vi "State-Space.vi"(0 "input points":dbl[](array[numeric]) format="%.2f", 1 "initial conditions":dbl[](array[numeric]) format="%.2f", 2 "MIMO state space":T1 {"D" format="%.2f"; "C" format="%.2f"; "B" format="%.2f"; "A" format="%.2f"}, 3 "dt":dbl=1e-09 min=1e-09 format="%.6f", 4 "initialize":bool) -> (5 "output points":dbl[](array[numeric]) format="%.2f", 6 "states":dbl[](array[numeric]) format="%.2f")   [LabVIEW 2020, in "NI_AdvCtrl_continuous linear.lvlib"]
doc: "LabVIEW no longer supports this VI. You can obtain similar functionality by installing the LabVIEW Simulation Module.\n\nCalculates the new output and the internal states, where the state-space representation, the initial condition, and the input vectors are given. The MIMO system is represented by dx(t)/dt=Ax(t)+Bu(t), y(t)=Cx(t)+Du(t)."
uses:
  <vilib>/addons/control/advanced/NI_AdvCtrl_continuous linear.lvlib
  <vilib>/addons/control/advanced/continuous linear.llb/Integrator (DBL Array).vi
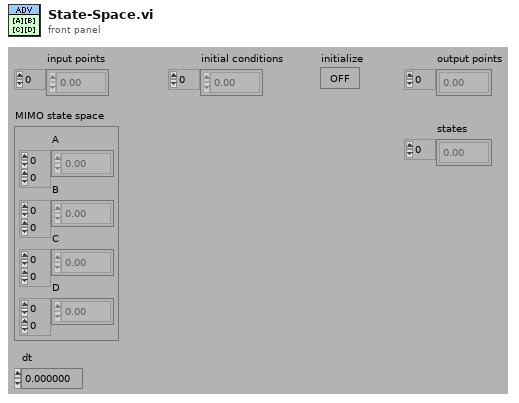
[diagram p1: front panel]
types:
  T1 = cluster{"A":dbl[][], "B":dbl[][], "C":dbl[][], "D":dbl[][]}
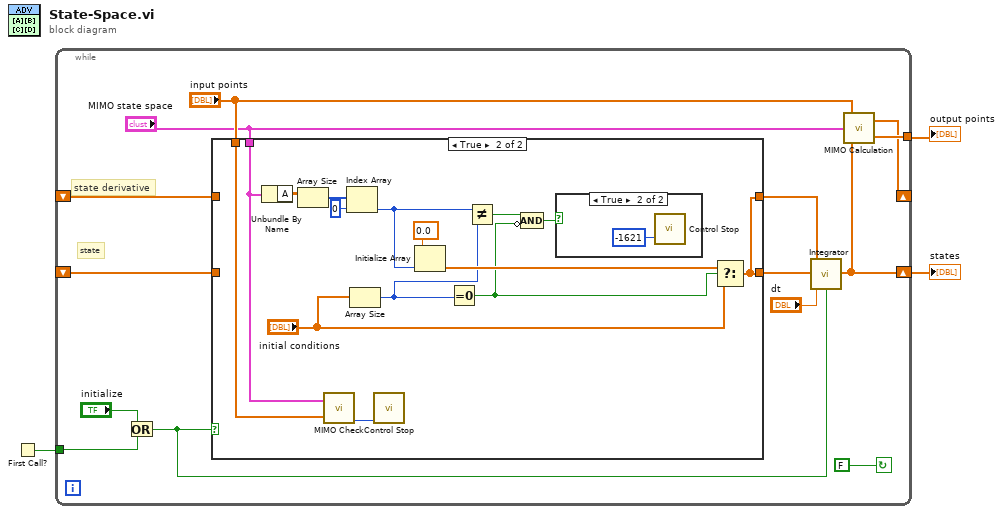
[diagram p0: block diagram]
diagram:
  n1 = First Call?() -> (First Call?: T/F=w1:bool)
  n2 = while {
    tunnel: w1 -> [w8]
    shift-left: _ -> [w14]
    shift-right: [w15] -> _
    tunnel: [w17] -> w3
    shift-left: _ -> [w16]
    shift-right: [w12] -> w2
    stop <- FALSE continue-if-true
    # "state"
    # "state derivative"
    n3 = Or(x="initialize", y=w8) -> (x .or. y?=w6:bool)
    n4 = case shown="True" w6 {
      tunnel: [w19 w20] -> w4
      tunnel: w16 -> [w19 _]
      tunnel: w14 -> [w18 _]
      tunnel: [w18 w20] -> w13
      tunnel: "input points" -> [_ w22]
      tunnel: "MIMO state space" -> [_ w28]
      frame False {
      }
      frame True {
        n5 = Unbundle By Name(w28) -> ("A"=w34:dbl[][])
        n6 = Array Size(array=w34) -> (size(s)=w32:i32[])
        n7 = call <vilib>:"MIMO Check.vi"("MIMO State-Space"=w28, "Input Points"=w22) -> ("error"=w27:i32)  [unwired: 3 out]
        n8 = Index Array(array=w32, index=0 ("Index")) -> (element=w21:i32)
        n9 = Array Size(array="initial conditions") -> (size(s)=w24:i32)
        n10 = call <vilib>:"Control Stop.vi"("error"=w27) -> ()  [unwired: 2 out]
        n11 = Initialize Array(0.0 ("Element Data"), w21) -> (w29:dbl[])
        n12 = Equal To 0?(x=w24) -> (x = 0?=w26:bool)
        n13 = Not Equal?(x=w21, y=w24) -> (x != y?=w25:bool)
        n14 = Compound Arithmetic op=AND(w25, invert w26) -> (w23:bool)
        n15 = case shown="True" w23 {
          frame False {
          }
          frame True {
            n16 = call <vilib>:"Control Stop.vi"("error"=-1621) -> ()  [unwired: 2 out]
          }
        }
        n17 = Select(t=w29, s=w26, f="initial conditions") -> (s? t:f=w20:dbl[])
      }
    }
    n18 = call-poly <vilib>:"Integrator.vi"("initialize"=w6, "dt"="dt", "initial conditions"=w4, "input points"=w13) -> ("output points"=w12:dbl[])  [unwired: 1 out]
    n19 = call <vilib>:"MIMO Calculation.vi"("x(n)"=w12, "MIMO State-Space"="MIMO state space", "u(n)"="input points") -> ("y(n)"=w17:dbl[], "x(n+1)"=w15:dbl[])
  }
  "output points" <- w3
  "states" <- w2
